vi "get_speed.vi"(8 "error in (no error)":errorcluster, 11 "SignalWriterMH110203USBStepperMotor in":refnum<class "SignalWriterMH110203USBStepperMotor.lvclass">) -> (0 "error out":errorcluster, 2 "speed":dbl, 3 "SignalWriterMH110203USBStepperMotor out":refnum<class "SignalWriterMH110203USBStepperMotor.lvclass">)   [LabVIEW 2010, in "SignalWriterMH110203USBStepperMotor.lvclass"]
uses:
  SignalWriterMH110203USBStepperMotor.lvclass
  SignalWriterMH110203USBStepperMotor.lvclass/SignalWriterMH110203USBStepperMotor.ctl
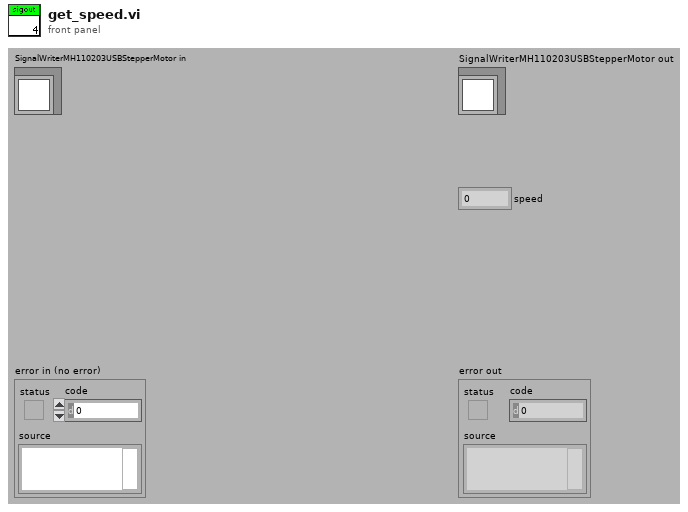
[diagram p1: front panel]
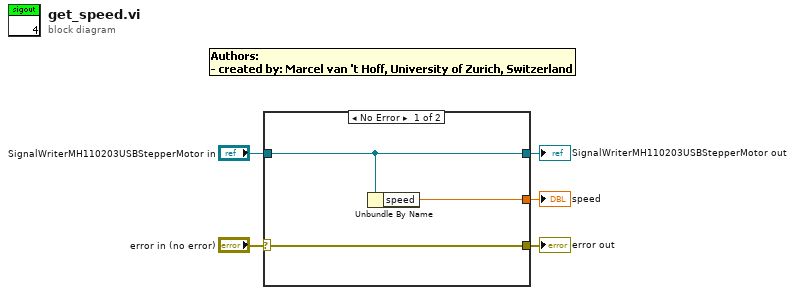
[diagram p0: block diagram]
diagram:
  n1 = case shown="No Error" "error in (no error)" {
    selector: "error in (no error)" -> [w8 w9]
    tunnel: [w8 w9] -> w4
    tunnel: [w7 w10] -> w2
    tunnel: "SignalWriterMH110203USBStepperMotor in" -> [w7 w10]
    tunnel: [w6 _] -> w1
    frame No Error {
      n2 = Unbundle By Name(w7) -> ("speed"=w6:dbl)
    }
    frame Error {
    }
  }
  "error out" <- w4
  "SignalWriterMH110203USBStepperMotor out" <- w2
  "speed" <- w1
